vi "Stop.vi"(4 "Time":dbl=1.0, 11 "error in":errorcluster) -> (3 "error out":errorcluster)   [LabVIEW 2015]
uses:
  References/Refnums.vi
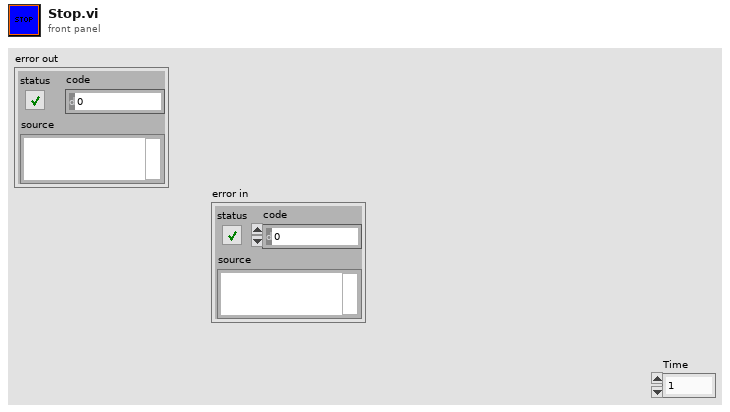
[diagram p1: front panel]
types:
  T1 = typedef "WPI_MotorControlDeviceRef.ctl" = cluster{"DeviceStatus":errorcluster, "Type":T2, "PWM":cluster{"PWM Channel":T3, "DeadBand":T4}, "CAN":cluster{"Device Number":u8, "Control Mode":T5, "Semaphore":T6, "Max Vout":dbl, "TalonSRX Control Mode":T7}, "Invert":bool}
  T2 = typedef "WPI_MotorControlType.ctl" = enum16{"PWM", "CAN", "CANTalonSRX"}
  T3 = typedef "FPGA_DIOPWMChannel.ctl" = enum8{"PWM 0", "PWM 1", "PWM 2", "PWM 3", "PWM 4", "PWM 5", "PWM 6", "PWM 7", "PWM 8", "PWM 9", "PWM MXP 0", "PWM MXP 1", "PWM MXP 2", "PWM MXP 3", "PWM MXP 4", "PWM MXP 5", "PWM MXP 6", "PWM MXP 7", "PWM MXP 8", "PWM MXP 9", "Invalid"}
  T4 = typedef "WPI_PWMDeadband.ctl" = cluster{"Name":string, "maxPositivePwm":i32, "minPositivePwm":i32, "centerPwm":i32, "maxNegativePwm":i32, "minNegativePwm":i32, "angularRange":u16}
  T5 = typedef "WPI_CANJaguar_ControlMode.ctl" = enum8{"Percent VBus", "Current", "Speed", "Position", "Voltage"}
  T6 = typedef "Semaphore RefNum" = refnum<k1>
  T7 = typedef "WPI_CANTalonSRX_APIControlMode.ctl" = enum8{"Percent VBus", "Speed", "Position", "Slave", "Unchanged / Invalid", "Voltage Compensation", "Current", "Motion Profile"}
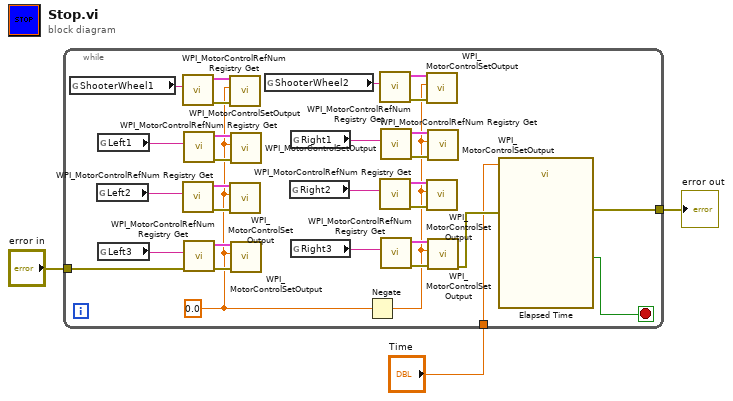
[diagram p0: block diagram]
diagram:
  n1 = while {
    tunnel: [w14] -> w3
    tunnel: "error in" -> [w13]
    tunnel: "Time" -> [w12]
    stop <- w16 stop-if-true
    w5 = 0.0 ("Output")
    n2 = global read "Refnums.vi" "ShooterWheel1"() -> (w9:string)
    n3 = global read "Refnums.vi" "Left2"() -> (w20:string)
    n4 = global read "Refnums.vi" "Left1"() -> (w19:string)
    n5 = global read "Refnums.vi" "Left3"() -> (w25:string)
    n6 = call <vilib>:"WPI_MotorControlRefNum Registry Get.vi"("refnum name"=w9) -> ("error out"=w11:errorcluster, "MotorControlDevRef"=w10:T1)  [unwired: 9 in]
    n7 = call <vilib>:"WPI_MotorControlRefNum Registry Get.vi"("refnum name"=w20) -> ("error out"=w22:errorcluster, "MotorControlDevRef"=w21:T1)  [unwired: 9 in]
    n8 = call <vilib>:"WPI_MotorControlRefNum Registry Get.vi"("refnum name"=w19) -> ("error out"=w17:errorcluster, "MotorControlDevRef"=w18:T1)  [unwired: 9 in]
    n9 = call <vilib>:"WPI_MotorControlRefNum Registry Get.vi"("error in (no error)"=w13, "refnum name"=w25) -> ("error out"=w23:errorcluster, "MotorControlDevRef"=w24:T1)  [unwired: 8 in]
    n10 = call <vilib>:"WPI_MotorControlSetOutput.vi"("error in (no error)"=w11, "Output"=w5, "MotorControlDevRef"=w10) -> ()  [unwired: 6 in, 3 out]
    n11 = call <vilib>:"WPI_MotorControlSetOutput.vi"("error in (no error)"=w22, "Output"=w5, "MotorControlDevRef"=w21) -> ()  [unwired: 6 in, 3 out]
    n12 = call <vilib>:"WPI_MotorControlSetOutput.vi"("error in (no error)"=w17, "Output"=w5, "MotorControlDevRef"=w18) -> ()  [unwired: 6 in, 3 out]
    n13 = call <vilib>:"WPI_MotorControlSetOutput.vi"("error in (no error)"=w23, "Output"=w5, "MotorControlDevRef"=w24) -> ()  [unwired: 6 in, 3 out]
    n14 = global read "Refnums.vi" "ShooterWheel2"() -> (w8:string)
    n15 = global read "Refnums.vi" "Right2"() -> (w31:string)
    n16 = global read "Refnums.vi" "Right1"() -> (w32:string)
    n17 = global read "Refnums.vi" "Right3"() -> (w26:string)
    n18 = Negate(x=w5) -> (-x=w4:dbl)
    n19 = call <vilib>:"WPI_MotorControlRefNum Registry Get.vi"("refnum name"=w8) -> ("error out"=w6:errorcluster, "MotorControlDevRef"=w7:T1)  [unwired: 9 in]
    n20 = call <vilib>:"WPI_MotorControlRefNum Registry Get.vi"("refnum name"=w31) -> ("error out"=w29:errorcluster, "MotorControlDevRef"=w30:T1)  [unwired: 9 in]
    n21 = call <vilib>:"WPI_MotorControlRefNum Registry Get.vi"("refnum name"=w32) -> ("error out"=w34:errorcluster, "MotorControlDevRef"=w33:T1)  [unwired: 9 in]
    n22 = call <vilib>:"WPI_MotorControlRefNum Registry Get.vi"("refnum name"=w26) -> ("error out"=w28:errorcluster, "MotorControlDevRef"=w27:T1)  [unwired: 9 in]
    n23 = call <vilib>:"WPI_MotorControlSetOutput.vi"("error in (no error)"=w6, "Output"=w4, "MotorControlDevRef"=w7) -> ()  [unwired: 6 in, 3 out]
    n24 = call <vilib>:"WPI_MotorControlSetOutput.vi"("error in (no error)"=w29, "Output"=w4, "MotorControlDevRef"=w30) -> ()  [unwired: 6 in, 3 out]
    n25 = call <vilib>:"WPI_MotorControlSetOutput.vi"("error in (no error)"=w34, "Output"=w4, "MotorControlDevRef"=w33) -> ()  [unwired: 6 in, 3 out]
    n26 = call <vilib>:"WPI_MotorControlSetOutput.vi"("error in (no error)"=w28, "Output"=w4, "MotorControlDevRef"=w27) -> ("error out"=w15:errorcluster)  [unwired: 6 in, 2 out]
    n27 = call "Elapsed Time"("Time Target (s)"=w12, "error in (no error)"=w15) -> ("Time has Elapsed"=w16:bool, "error out"=w14:errorcluster)  [unwired: 10 in, 6 out]
  }
  "error out" <- w3
